vi "Set Ramp Rate Units.vi"(2 "error in":T1, 3 "Ramp Rate Units":u16(ring) items=["Per SECOND", "Per MINUTE"], 4 "VISA resource name":refnum<visa-resource-name>) -> (0 "error out":T1, 1 "VISA resource name out":refnum<visa-resource-name>)   [LabVIEW 2019]
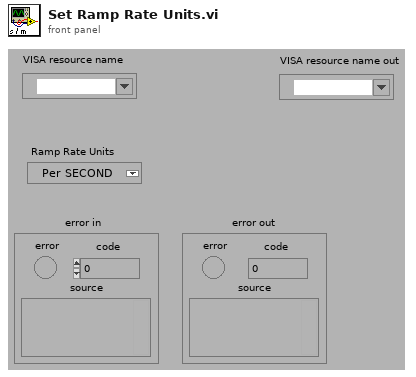
[diagram p1: front panel]
types:
  T1 = cluster{"error":bool, "code":i32, "source":string}
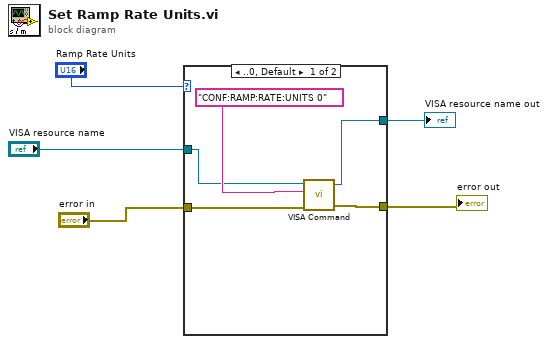
[diagram p0: block diagram]
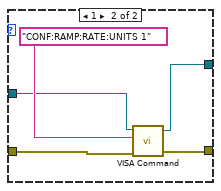
[diagram p2: hidden frame]
diagram:
  n1 = case shown="..0, Default" "Ramp Rate Units" {
    tunnel: "error in" -> [w9 w14]
    tunnel: [w8 w13] -> w3
    tunnel: "VISA resource name" -> [w7 w12]
    tunnel: [w6 w11] -> w1
    frame ..0, Default {
      n2 = call "VISA Command.vi"("error in (no error)"=w9, "Command"="CONF:RAMP:RATE:UNITS 0", "VISA resource name"=w7) -> ("error out"=w8:errorcluster, "VISA resource name out"=w6:refnum<visa-resource-name>)  [unwired: 1 in, 1 out]
    }
    frame 1 {
      n3 = call "VISA Command.vi"("error in (no error)"=w14, "Command"="CONF:RAMP:RATE:UNITS 1", "VISA resource name"=w12) -> ("error out"=w13:errorcluster, "VISA resource name out"=w11:refnum<visa-resource-name>)  [unwired: 1 in, 1 out]
    }
  }
  "error out" <- w3
  "VISA resource name out" <- w1
